vi "Fetch Single Record.vi"(0 "device session in":refnum<class "Device Session.lvclass">, 1 "starting record":u64, 5 "fetch relative to":T3=enum."First Pretrigger Sample", 7 "number of samples":u64=1000, 9 "timeout (ms)":i32=1000, 11 "error in":errorcluster, 12 "fetch offset":i64, 13 "Chan#":T1=enum."1") -> (4 "device session out":refnum<class "Device Session.lvclass">, 6 "data":dbl[][](array[numeric]), 8 "relativeX (samples)":dbl, 14 "requested record info":T2={"number of samples"=0, "starting sample number"=0, "number of channels"=1, "timestamps"=[]}, 15 "error out":errorcluster)   [LabVIEW 2021, in "Device Session.lvclass"]
doc: "Fetches data from a single record in an acquisition. No data is returned if this VI times out. You must run the <B>Initiate</B> VI before running this VI.\n\n<B>Input Parameters</B>\n\n<B>device session in</B> is a reference to the Device Session object, which contains a session to each instrument design library used in this sample project. This parameter is obtained from the 'Open Session' VI.\n\n<B>starting record</B> specifies the record to retrieve. Index of the record numbers starts at 0.\n\n<B>fetch relative to</B> specifies the relative location within the acquired record from where the VI begins to fetch data.\n\n'First Sample': the fetch starts at the first sample acquired by the device. If the device wraps data in its memory buffer, the first sample is no longer available. In this case, the VI returns an error if 'fetch offset' specifies a location that is within the overwritten portion of the memory buffer.\n'Reference Trigger Sample': the fetch starts relative to the Reference Trigger.\n'First Pretrigger Sample': the fetch starts relative to the first pretrigger sample acquired. If you do not configure a Reference Trigger, 'First Pretrigger Sample' behaves the same as 'First Sample' because there are no pretrigger samples.\n'Most Recent Sample': the fetch starts relative to the most recently acquired sample. The value of 'fetch offset' must be negative. This VI doesn't support this option. Consider using the 'Fetch Single Record' VI instead.\n'Current Read Position': the fetch starts after the last fetched sample. This VI doesn't support this option. Consider using the 'Fetch Single Record' VI instead.\n\n<B>number of samples</B> specifies the number of samples to fetch. The default value is 1000.\n\n<B>timeout (ms)</B> specifies the time, in milliseconds, allotted for the Fetch Multiple Records VI to complete execution of each record before returning a timeout error. A value of -1 specifies that the VI waits until all data is available. A value of 0 is not supported. The default value is 10,000. You cannot abort a pending fetch using the Abort VI or Close VI.\n\n<B>fetch offset</B> specifies the offset relative to the position, which is specified by the 'fetch relative to' parameter, from which to start fetching data. Offset can be a positive or negative value. The default value is 0.\n\n<B>error in</B> describes error conditions that occur before this node runs. This input provides standard 'error in' functionality.\n\n<B>Output Parameters</B>\n\n<B>device session out</B> passes a reference to the session to the next VI.\n\n<B>data</B> returns the fetched data.\n\n<B>requested record info</B> returns the record parameters configuration.\n\n<B>relativeX (samples)</B> returns the relative position from the trigger to the first sample in the acquired data.\n\n<B>error out</B> contains error information. This output provides standard 'error out' functionality."
uses:
  Device Session.lvclass
  <instrlib>/_niInstr/Multirecord Acquisition/Interface/v1/Host/Public/Fetch Relative To Enum.ctl
  <instrlib>/_niInstr/Multirecord Acquisition/Interface/v1/Host/Public/Requested Record Info.ctl
  Enums/Channel Numbers.ctl
  Device Session.lvclass/Device Session.ctl
  <instrlib>/_niInstr/Multirecord Acquisition/Interface/v1/Host/Private/Fetch Single Record DBL NCh Wrapper.vi
  <instrlib>/HSAI-RIO/Config/Group A/v1/Host/Main/niHSAI Group A Config v1 Host.lvclass
  <instrlib>/_niInstr/Multirecord Acquisition/Interface/v1/Host/niInstr Multirecord Acquisition v1 Host.lvclass
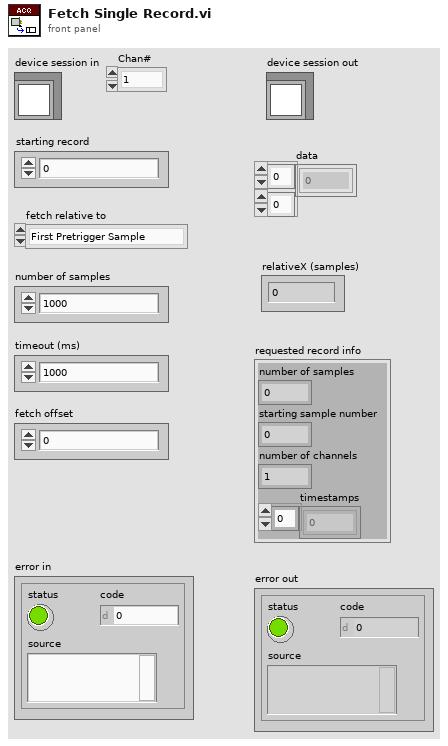
[diagram p1: front panel]
types:
  T1 = typedef "Channel Numbers.ctl" = enum16{"0", "1", "2", "3", "4", "5", "6", "7"}
  T2 = typedef "niInstr Multirecord Acquisition v1 Host.lvclass/Requested Record Info.ctl" = cluster{"number of samples":u64, "starting sample number":u64, "number of channels":u64, "timestamps":u64[]}
  T3 = typedef "niInstr Multirecord Acquisition v1 Host.lvclass/Fetch Relative To Enum.ctl" = enum16{"First Sample", "Reference Trigger Sample", "First Pretrigger Sample", "Most Recent Sample", "Current Read Position"}
  T4 = typedef "Device Session.lvclass/Device Session Object.ctl" = cluster{"fpga reference":T5, "reg bus":refnum<class "niInstr FIFO Register Bus v1 Host.lvclass">, "subsystem map":refnum<class "niInstr Subsystem Map v1 Host.lvclass">, "cal data":refnum<class "niHSAI Cal Data v1 Host.lvclass">, "config":refnum<class "niHSAI Group A Config v1 Host.lvclass">, "acquisition 0":refnum<class "niInstr Multirecord Acquisition v1 Host.lvclass">, "acquisition 1":refnum<class "niInstr Multirecord Acquisition v1 Host.lvclass">, "acquisition 2":refnum<class "niInstr Multirecord Acquisition v1 Host.lvclass">, "acquisition 3":refnum<class "niInstr Multirecord Acquisition v1 Host.lvclass">, "acquisition 4":refnum<class "niInstr Multirecord Acquisition v1 Host.lvclass">, "acquisition 5":refnum<class "niInstr Multirecord Acquisition v1 Host.lvclass">, "acquisition 6":refnum<class "niInstr Multirecord Acquisition v1 Host.lvclass">, "acquisition 7":refnum<class "niInstr Multirecord Acquisition v1 Host.lvclass">, "number of selected acq channels":u8, "selected acq channels":bool[], "number of channels":u32, "configured channels":bool[], "acq configuration":cluster{"number of samples":u64, "number of records":u64, "pretrigger samples":u64}, "actual channel configuration":T6[], "sample clock rate (Hz)":dbl, "scaling coefficients":T10[]}
  T5 = typedef "Device Session.lvclass/FPGA Refnum.ctl" = refnum<k20>
  T6 = typedef "niHSAI Types v1 Host.lvlib/Channel Configuration.ctl" = cluster{"channel":u32, "coupling":T7, "impedance":T8, "bandwidth":T9, "vertical range":dbl, "vertical offset":dbl}
  T7 = typedef "niHSAI Types v1 Host.lvlib/Coupling.ctl" = enum8{"Default", "DC", "AC"}
  T8 = typedef "niHSAI Types v1 Host.lvlib/Impedance.ctl" = enum8{"Default", "1 mega ohm", "50 ohm"}
  T9 = typedef "niHSAI Types v1 Host.lvlib/Bandwidth.ctl" = enum8{"Default", "Full Bandwidth", "Anti-alias Filter", "150 MHz"}
  T10 = typedef "niInstr Multirecord Acquisition v1 Host.lvclass/Scaling Coefficient.ctl" = cluster{"gain":dbl, "offset":dbl}
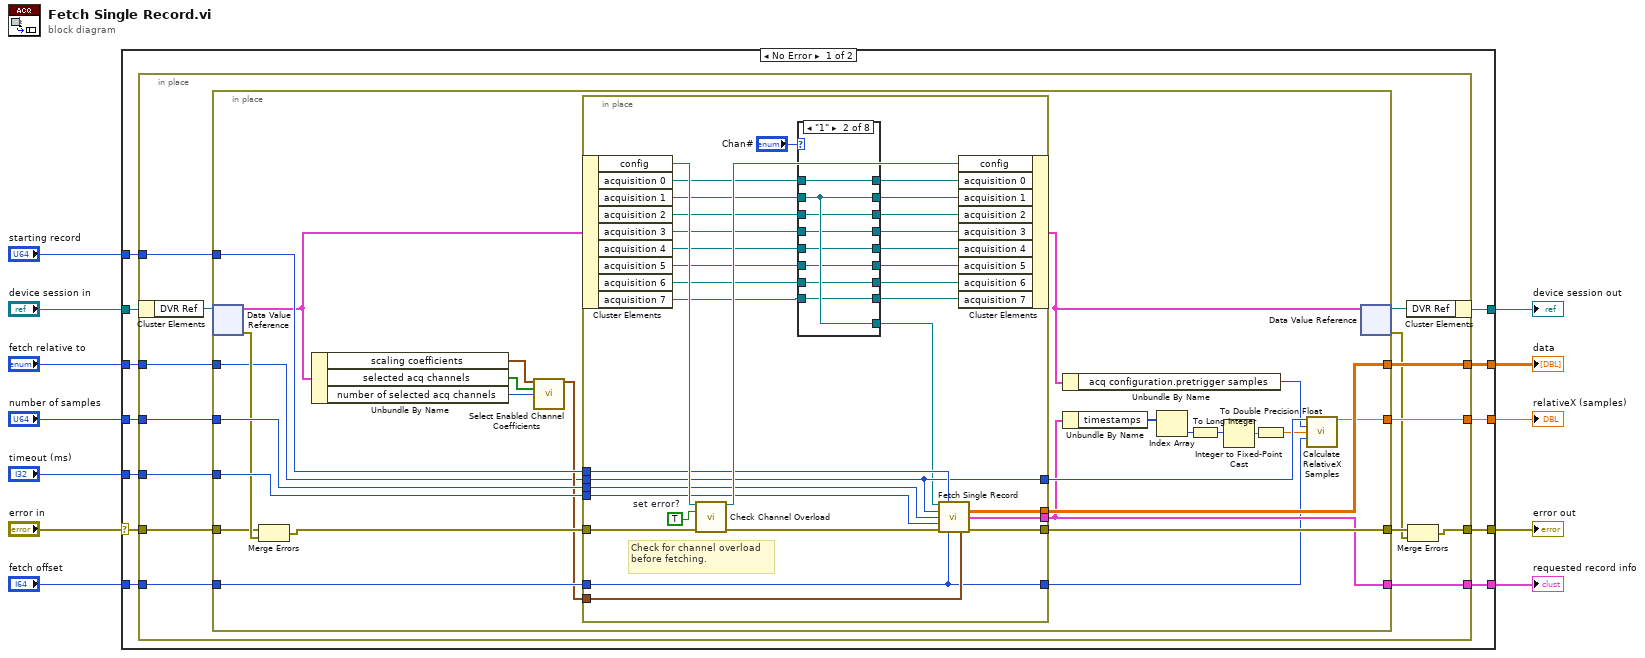
[diagram p0: block diagram]
diagram:
  n1 = case shown="No Error" "error in" {
    selector: "error in" -> [w24 w162]
    tunnel: [w19 w162] -> w11
    tunnel: "device session in" -> [w14 w161]
    tunnel: [w13 w161] -> w9
    tunnel: "number of samples" -> [w23 _]
    tunnel: "timeout (ms)" -> [w22 _]
    tunnel: "fetch offset" -> [w21 _]
    tunnel: "starting record" -> [w20 _]
    tunnel: "fetch relative to" -> [w18 _]
    tunnel: [w17 _] -> w3
    tunnel: [w16 _] -> w1
    tunnel: [w15 _] -> w2
    frame No Error {
      n2 = in-place {
        in-place-border: w24 -> [w38]
        in-place-border: w23 -> [w37]
        in-place-border: w22 -> [w36]
        in-place-border: w21 -> [w35]
        in-place-border: w20 -> [w34]
        in-place-border: [w33] -> w19
        in-place-border: w18 -> [w31]
        in-place-border: [w30] -> w17
        in-place-border: [w29] -> w16
        in-place-border: [w28] -> w15
        n3 = in-place-cluster #1(w14) -> ("DVR Ref"=w26:refnum<data-value>)
        n4 = in-place {
          in-place-border: w38 -> [w60]
          in-place-border: [w64] -> w32
          in-place-border: w37 -> [w63]
          in-place-border: w36 -> [w62]
          in-place-border: w35 -> [w48]
          in-place-border: w34 -> [w57]
          in-place-border: w31 -> [w45]
          in-place-border: [w56] -> w30
          in-place-border: [w55] -> w29
          in-place-border: [w43] -> w28
          n5 = in-place-dvr #2(w26) -> (w46:T4, w61:errorcluster)
          n6 = Merge Errors(w60, w61) -> (w49:errorcluster)
          n7 = Unbundle By Name(w46) -> ("scaling coefficients"=w54:T10[], "selected acq channels"=w59:bool[], "number of selected acq channels"=w58:u8)
          n8 = call "Select Enabled Channel Coefficients.vi"("configured scaling coefficients"=w54, "selected acq channels to store"=w59, "number of selected acq channels to store"=w58) -> ("stored scaling coefficients"=w47:T10[])  [unwired: 12 in]
          n9 = in-place {
            in-place-border: [w96] -> w64
            in-place-border: w63 -> [w86]
            in-place-border: w62 -> [w85]
            in-place-border: w57 -> [w87]
            in-place-border: [w93] -> w56
            in-place-border: [w92] -> w43
            in-place-border: w49 -> [w91]
            in-place-border: w45 -> [w84]
            in-place-border: w48 -> [w83]
            in-place-border: w47 -> [w90]
            in-place-border: [w84] -> w44
            in-place-border: [w83] -> w42
            w94 = TRUE  # set error?
            # "Check for channel overload before fetching."
            n10 = in-place-cluster #3(w46) -> ("config"=w89:refnum<class "niHSAI Group A Config v1 Host.lvclass">, "acquisition 0"=w81:refnum<class "niInstr Multirecord Acquisition v1 Host.lvclass">, "acquisition 1"=w80:refnum<class "niInstr Multirecord Acquisition v1 Host.lvclass">, "acquisition 2"=w79:refnum<class "niInstr Multirecord Acquisition v1 Host.lvclass">, "acquisition 3"=w78:refnum<class "niInstr Multirecord Acquisition v1 Host.lvclass">, "acquisition 4"=w77:refnum<class "niInstr Multirecord Acquisition v1 Host.lvclass">, "acquisition 5"=w76:refnum<class "niInstr Multirecord Acquisition v1 Host.lvclass">, "acquisition 6"=w75:refnum<class "niInstr Multirecord Acquisition v1 Host.lvclass">, "acquisition 7"=w74:refnum<class "niInstr Multirecord Acquisition v1 Host.lvclass">)
            n11 = call-dynamic "Check Channel Overload.vi"("session in"=w89, "set error? (T)"=w94, "error in"=w91) -> ("session out"=w88:refnum<class "niHSAI Group A Config v1 Host.lvclass">, "error out"=w95:errorcluster)  [unwired: 10 in, 1 out]
            n12 = case shown="\"1\"" "Chan#" {
              tunnel: w81 -> [w104 w111 w119 w127 w135 w143 w151 w159]
              tunnel: w80 -> [w103 w112 w118 w126 w134 w142 w150 w158]
              tunnel: [w104 w112 w120 w128 w136 w144 w152 w160] -> w66
              tunnel: w79 -> [w102 w110 w120 w125 w133 w141 w149 w157]
              tunnel: w78 -> [w101 w109 w117 w128 w132 w140 w148 w156]
              tunnel: w77 -> [w100 w108 w116 w124 w136 w139 w147 w155]
              tunnel: w76 -> [w99 w107 w115 w123 w131 w144 w146 w154]
              tunnel: w75 -> [w98 w106 w114 w122 w130 w138 w152 w153]
              tunnel: w74 -> [w97 w105 w113 w121 w129 w137 w145 w160]
              tunnel: [w104 w111 w119 w127 w135 w143 w151 w159] -> w65
              tunnel: [w103 w112 w118 w126 w134 w142 w150 w158] -> w73
              tunnel: [w102 w110 w120 w125 w133 w141 w149 w157] -> w72
              tunnel: [w101 w109 w117 w128 w132 w140 w148 w156] -> w71
              tunnel: [w100 w108 w116 w124 w136 w139 w147 w155] -> w70
              tunnel: [w99 w107 w115 w123 w131 w144 w146 w154] -> w69
              tunnel: [w98 w106 w114 w122 w130 w138 w152 w153] -> w68
              tunnel: [w97 w105 w113 w121 w129 w137 w145 w160] -> w67
              frame "0" {
              }
              frame "1" {
              }
              frame "2" {
              }
              frame "3" {
              }
              frame "4" {
              }
              frame "5" {
              }
              frame "6" {
              }
              frame "7" {
              }
            }
            n13 = call-poly <instrlib>:"Fetch Single Record.vi"("session in"=w66, "record number"=w87, "fetch relative to"=w84, "number of samples"=w86, "timeout (ms)"=w85, "error in"=w95, "fetch offset"=w83, "scaling coefficients"=w90) -> ("data"=w93:dbl[][], "requested record info"=w92:T2, "error out"=w96:errorcluster)  [unwired: 4 in, 1 out]
            n14 = in-place-cluster #3("config"=w88, "acquisition 0"=w65, "acquisition 1"=w73, "acquisition 2"=w72, "acquisition 3"=w71, "acquisition 4"=w70, "acquisition 5"=w69, "acquisition 6"=w68, "acquisition 7"=w67) -> (w40:T4)
          }
          n15 = Unbundle By Name(w40) -> ("acq configuration.pretrigger samples"=w39:u64)
          n16 = Unbundle By Name(w43) -> ("timestamps"=w51:u64[])
          n17 = Index Array(array=w51) -> (element=w50:u64)  [unwired: 1 in]
          n18 = To Long Integer(number=w50) -> (32bit integer=w52:i32)
          n19 = Integer to Fixed-Point Cast(integer=w52) -> (fixed-point=w53:fxp<+/-,32,5>)  [unwired: 1 in]
          n20 = To Double Precision Float(number=w53) -> (double precision float=w41:dbl)
          n21 = call "Calculate RelativeX Samples.vi"("fetch relative to"=w44, "pretrigger samples"=w39, "timestamps"=w41, "fetch offset"=w42) -> ("relativeX (samples)"=w55:dbl)  [unwired: 11 in]
          n22 = in-place-dvr #2(w40) -> (w25:refnum<data-value>, w27:errorcluster)
        }
        n23 = in-place-cluster #1("DVR Ref"=w25) -> (w13:refnum<class "Device Session.lvclass">)
        n24 = Merge Errors(w32, w27) -> (w33:errorcluster)
      }
    }
    frame Error {
    }
  }
  "error out" <- w11
  "device session out" <- w9
  "data" <- w3
  "requested record info" <- w2
  "relativeX (samples)" <- w1
